vi "Wait for pump.vi"(8 "error in (no error)":errorcluster, 11 "pump":enum16{"MAIN_PUMP"}(ring)) -> (0 "error out":errorcluster)   [LabVIEW 2018, in "cetoni.lvlib" / "cetoni.lvclass"]
uses:
  cetoni.lvclass
  Resources/GLOBAL/GLOBAL Time-critical.vi
  <userlib>/QmixLib/QmixLib.lvlib
  Program Files/cetoni/QmixSDK/lib/labview/labbCAN_Pump_API/labbCAN_Pump_API.lvlib
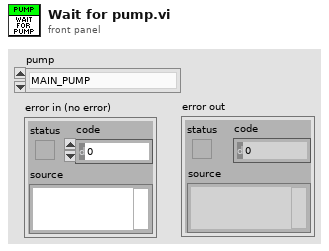
[diagram p1: front panel]
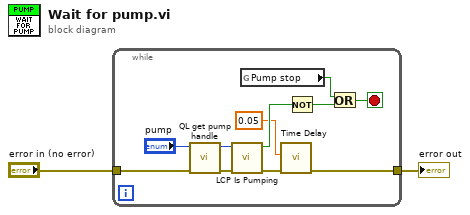
[diagram p0: block diagram]
diagram:
  n1 = while {
    tunnel: [w10] -> w1
    tunnel: "error in (no error)" -> [w9]
    stop <- w7 stop-if-true
    n2 = call <userlib>:"QL get pump handle.vi"("error in (no error)"=w9, "pump"="pump") -> ("error out"=w13:errorcluster, "pump handle"=w12:u64)  [unwired: 8 in]
    n3 = call "LCP Is Pumping.vi"("error in (no error)"=w13, "Pump Handle"=w12) -> ("error out"=w11:errorcluster, "Is pumping"=w6:bool)  [unwired: 8 in]
    n4 = global read "GLOBAL Time-critical.vi" "Pump stop"() -> (w4:bool)
    n5 = call "Time Delay"("error in (no error)"=w11, "Delay Time (s)"=0.05) -> ("error out"=w10:errorcluster)  [unwired: 9 in]
    n6 = Not(x=w6) -> (.not. x?=w5:bool)
    n7 = Or(x=w4, y=w5) -> (x .or. y?=w7:bool)
  }
  "error out" <- w1
